vi "Main.vi"(8 "error in":errorcluster, 11 "gRPC Server Tester in":refnum<class "gRPC Server Tester.lvclass">) -> (0 "error out":errorcluster, 3 "gRPC Server Tester out":refnum<class "gRPC Server Tester.lvclass">)   [LabVIEW 2019, in "gRPC Server Tester.lvclass"]
doc: "The <b>Queued Message Handler</b> of the Worker that owns this VI."
uses:
  gRPC Server Tester.lvclass
  C:/Program Files (x86)/National Instruments/LabVIEW 2019/vi.lib/addons/_Workers/Library/Classes/Worker/Worker.lvclass
  Generated_server/RPC Messages/w4lvgrpc_Msg_ToClient_4.ctl
  Generated_server/RPC Messages/w4lvgrpc_Msg_ToClient_1.ctl
  Generated_server/RPC Messages/w4lvgrpc_Msg_ToClient_2.ctl
  Generated_server/RPC Messages/w4lvgrpc_Msg_ToClient_3.ctl
  Generated_server/RPC Messages/w4lvgrpc_Msg_ToClient_5.ctl
  Generated_server/RPC Messages/w4lvgrpc_Msg_ToServer_1.ctl
  Generated_server/RPC Messages/w4lvgrpc_Msg_ToServer_2.ctl
  Generated_server/RPC Messages/w4lvgrpc_Msg_ToServer_3.ctl
  Generated_server/RPC Messages/w4lvgrpc_Msg_ToServer_4.ctl
  Generated_server/RPC Messages/w4lvgrpc_Msg_ToServer_5.ctl
  gRPC Server Tester.lvclass/gRPC Server Tester.ctl
  gRPC Server/gRPC Server/rqp_Msg_ToClient_1.ctl
  gRPC Server/gRPC Server/rqp_Msg_ToClient_2.ctl
  gRPC Server/gRPC Server/rqp_Msg_ToClient_3.ctl
  gRPC Server/gRPC Server/rqp_Msg_ToClient_4.ctl
  gRPC Server/gRPC Server/rqp_Msg_ToClient_5.ctl
  Initialization Data.ctl
  Response Cases.ctl
  rql_Create gRPC Server.ctl
  gRPC Server/gRPC Server/rwr_Create gRPC Server.ctl
  rql_Destroy gRPC Server.ctl
  <vilib>/addons/_Workers/Library/Classes/Message Queue/Message Queue.lvclass
  gRPC Server/gRPC Server/gRPC Server.lvclass
  Generated_server/Generated_server.lvlib
panel:
  out "Msg_ToServer_5":T1
  out "Msg_ToServer_4":T2
  out "Msg_ToServer_3":T3
  out "Msg_ToServer_2":T4
  out "Msg_ToServer_1":T5
  in  "Msg_ToClient_5":T6
  in  "Msg_ToClient_3":T7
  in  "Msg_ToClient_2":T8
  in  "Msg_ToClient_1":T9
  in  "Msg_ToClient_4":T10
  out "Client ID":u64
  out "Client Connected":bool
  out "Listening Port":i32
  out "Server Listening":bool
  in  "Server Address":string="localhost:50070"
  in  "Destroy gRPC Server":bool
  in  "Create gRPC Server":bool
  # "gRPC Server Worker - Public Requests"
  # "Messages Server -> Client"
  # "gRPC Server Worker Template Example"
  # "Instructions:\n\nSee project file called Readme.md"
  # "gRPC Server Worker - Public Responses"
  # "Messages Client -> Server"
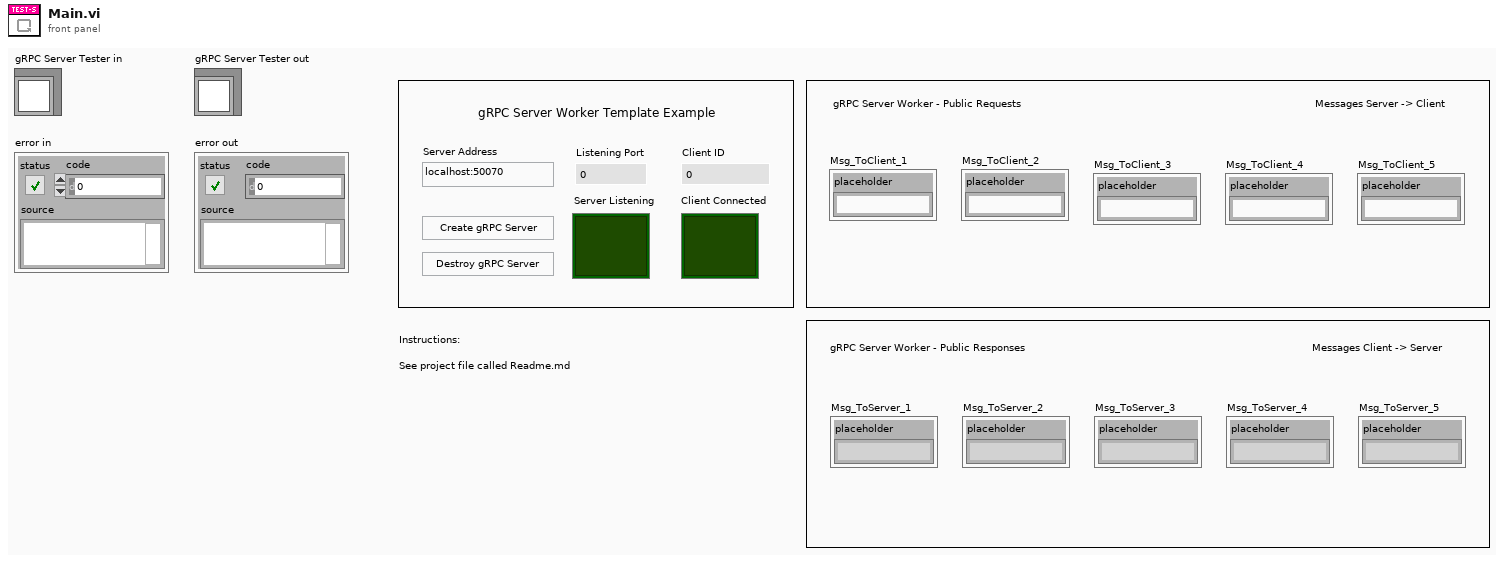
[diagram p1: front panel]
types:
  T1 = typedef "Generated_server.lvlib/w4lvgrpc_Msg_ToServer_5.ctl" = cluster{"placeholder":string}
  T2 = typedef "Generated_server.lvlib/w4lvgrpc_Msg_ToServer_4.ctl" = cluster{"placeholder":string}
  T3 = typedef "Generated_server.lvlib/w4lvgrpc_Msg_ToServer_3.ctl" = cluster{"placeholder":string}
  T4 = typedef "Generated_server.lvlib/w4lvgrpc_Msg_ToServer_2.ctl" = cluster{"placeholder":string}
  T5 = typedef "Generated_server.lvlib/w4lvgrpc_Msg_ToServer_1.ctl" = cluster{"placeholder":string}
  T6 = typedef "Generated_server.lvlib/w4lvgrpc_Msg_ToClient_5.ctl" = cluster{"placeholder":string}
  T7 = typedef "Generated_server.lvlib/w4lvgrpc_Msg_ToClient_3.ctl" = cluster{"placeholder":string}
  T8 = typedef "Generated_server.lvlib/w4lvgrpc_Msg_ToClient_2.ctl" = cluster{"placeholder":string}
  T9 = typedef "Generated_server.lvlib/w4lvgrpc_Msg_ToClient_1.ctl" = cluster{"placeholder":string}
  T10 = typedef "Generated_server.lvlib/w4lvgrpc_Msg_ToClient_4.ctl" = cluster{"placeholder":string}
  T11 = typedef "gRPC Server Tester.lvclass/Initialization Data.ctl" = cluster{"Response Cases":T12}
  T12 = typedef "gRPC Server Tester.lvclass/Response Cases.ctl" = cluster{"Placeholder - Can be deleted":string}
  T13 = typedef "gRPC Server Tester.lvclass/rql_Create gRPC Server.ctl" = cluster{"String":string}
  T14 = typedef "gRPC Server (template.proto).lvlib/gRPC Server.lvclass/rwr_Create gRPC Server.ctl" = cluster{"Server Key File (.key)":path, "Server Certificate File (.crt)":path, "Server Address":string}
  T15 = typedef "gRPC Server Tester.lvclass/rql_Destroy gRPC Server.ctl" = cluster{"String":string}
  T16 = typedef "gRPC Server (template.proto).lvlib/gRPC Server.lvclass/rqp_Msg_ToClient_1.ctl" = cluster{"w4lvgrpc_Msg_ToClient_1":T9}
  T17 = typedef "gRPC Server (template.proto).lvlib/gRPC Server.lvclass/rqp_Msg_ToClient_2.ctl" = cluster{"w4lvgrpc_Msg_ToClient_2":T8}
  T18 = typedef "gRPC Server (template.proto).lvlib/gRPC Server.lvclass/rqp_Msg_ToClient_3.ctl" = cluster{"w4lvgrpc_Msg_ToClient_3":T7}
  T19 = typedef "gRPC Server (template.proto).lvlib/gRPC Server.lvclass/rqp_Msg_ToClient_4.ctl" = cluster{"w4lvgrpc_Msg_ToClient_4":T10}
  T20 = typedef "gRPC Server (template.proto).lvlib/gRPC Server.lvclass/rqp_Msg_ToClient_5.ctl" = cluster{"w4lvgrpc_Msg_ToClient_5":T6}
  T21 = typedef "gRPC Server (template.proto).lvlib/gRPC Server.lvclass/rwr_Create gRPC Server Reply.ctl" = cluster{"Listening Port":i32}
  T22 = typedef "gRPC Server (template.proto).lvlib/gRPC Server.lvclass/rsp_Connection Notify.ctl" = cluster{"gRPC ID":T23, "Connected?":bool}
  T23 = typedef "grpc-lvsupport-release.lvlib/grpcId.ctl" = u64
  T24 = typedef "gRPC Server (template.proto).lvlib/gRPC Server.lvclass/rsp_Server Error.ctl" = errorcluster
  T25 = typedef "gRPC Server (template.proto).lvlib/gRPC Server.lvclass/rsp_Msg_ToServer_1.ctl" = cluster{"w4lvgrpc_Msg_ToServer_1":T5}
  T26 = typedef "gRPC Server (template.proto).lvlib/gRPC Server.lvclass/rsp_Msg_ToServer_2.ctl" = cluster{"w4lvgrpc_Msg_ToServer_2":T4}
  T27 = typedef "gRPC Server (template.proto).lvlib/gRPC Server.lvclass/rsp_Msg_ToServer_3.ctl" = cluster{"w4lvgrpc_Msg_ToServer_3":T3}
  T28 = typedef "gRPC Server (template.proto).lvlib/gRPC Server.lvclass/rsp_Msg_ToServer_4.ctl" = cluster{"w4lvgrpc_Msg_ToServer_4":T2}
  T29 = typedef "gRPC Server (template.proto).lvlib/gRPC Server.lvclass/rsp_Msg_ToServer_5.ctl" = cluster{"w4lvgrpc_Msg_ToServer_5":T1}
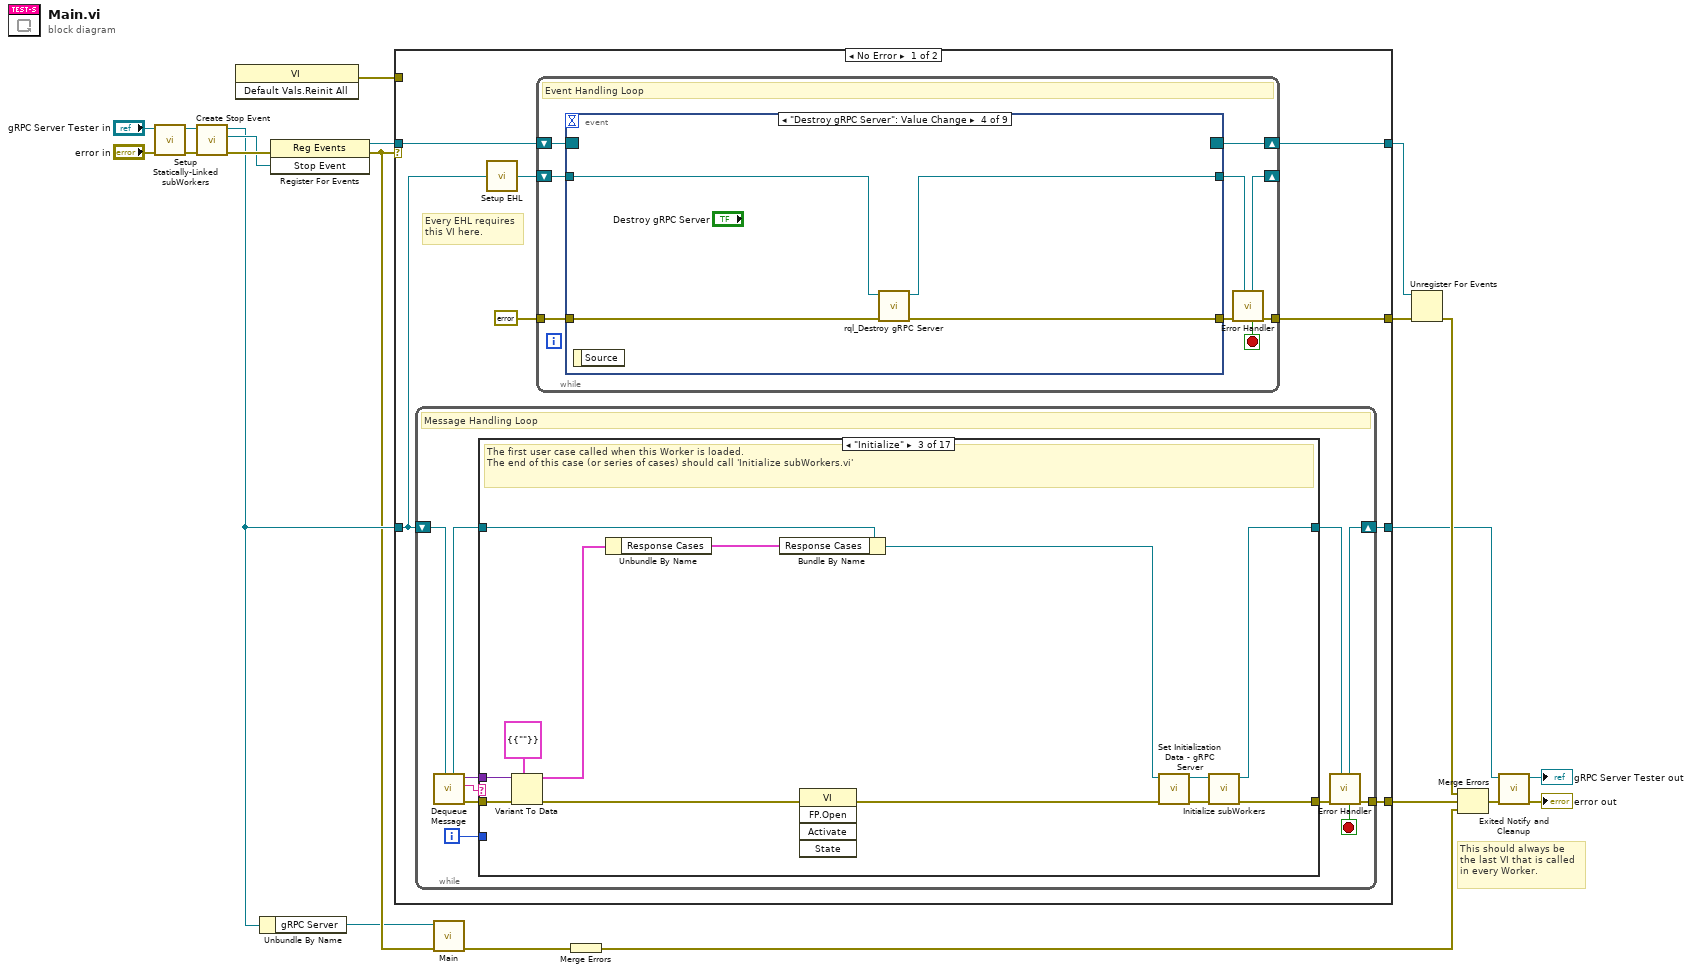
[diagram p0: block diagram]
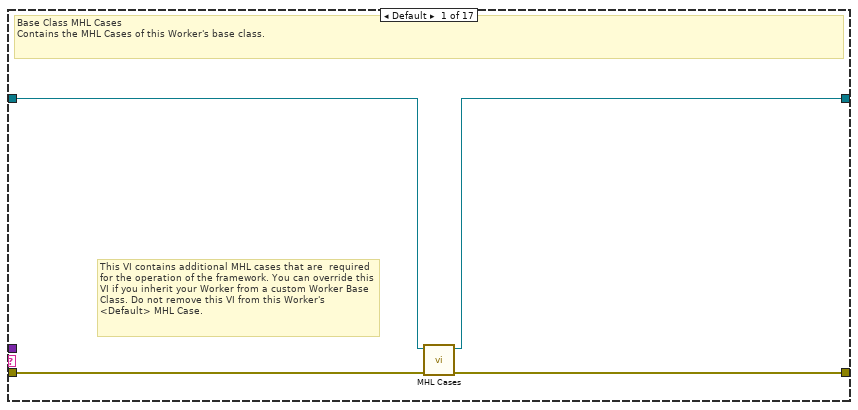
[diagram p2: hidden frame]
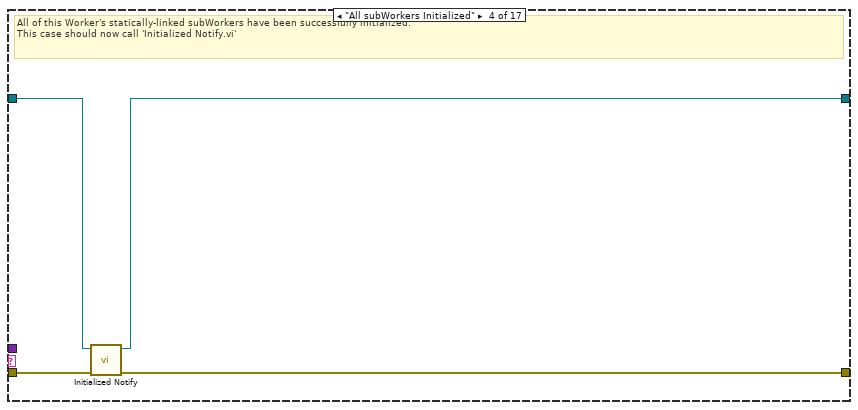
[diagram p4: hidden frame]
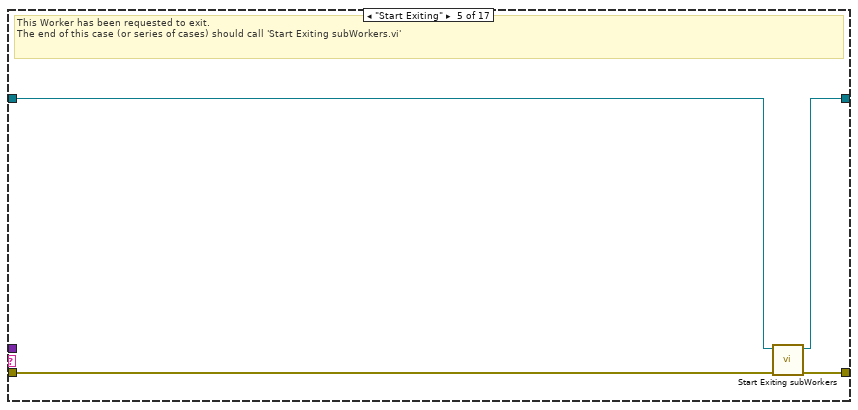
[diagram p5: hidden frame]
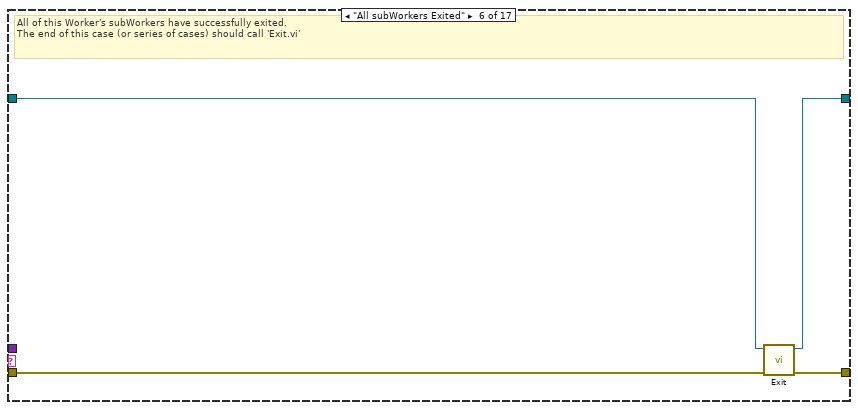
[diagram p6: hidden frame]
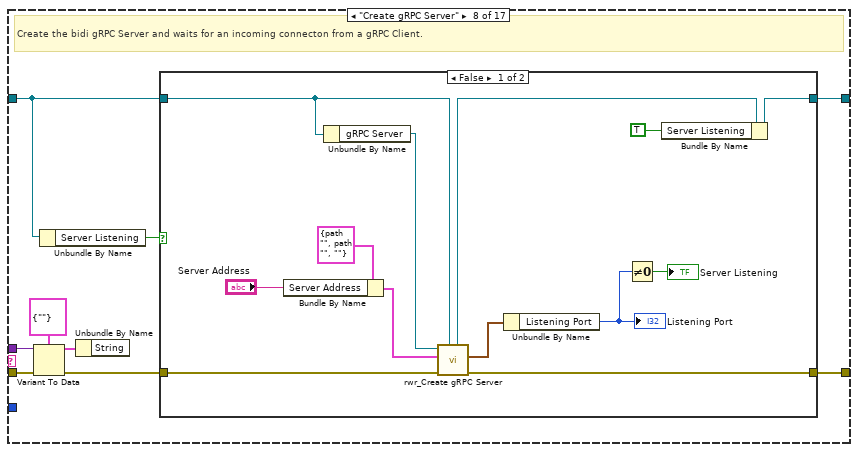
[diagram p8: hidden frame]
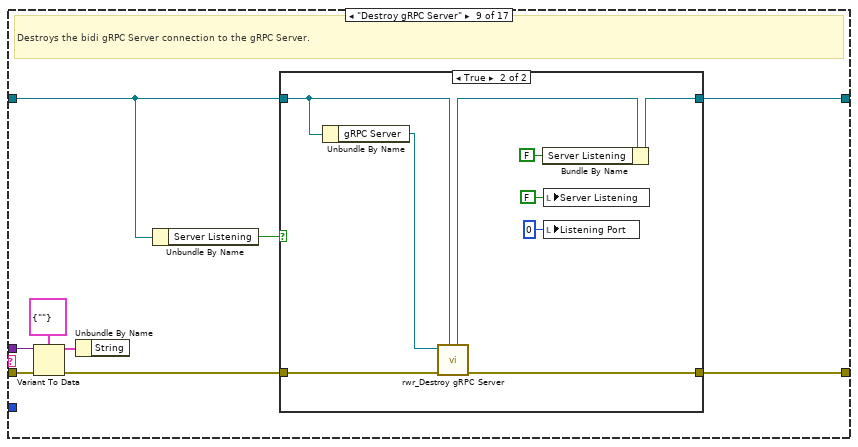
[diagram p10: hidden frame]
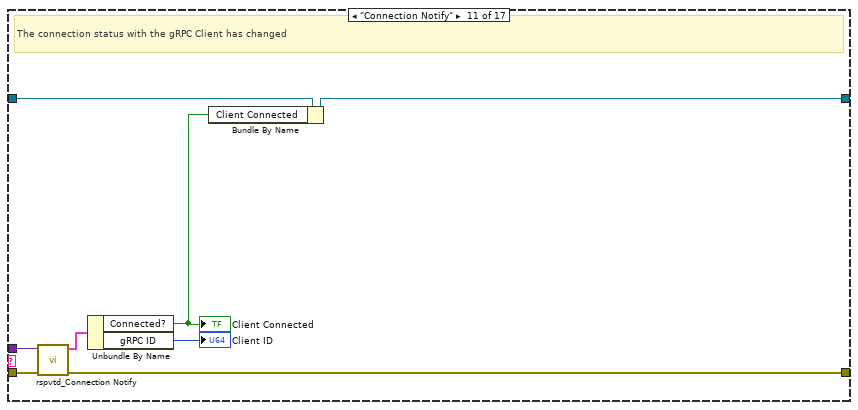
[diagram p13: hidden frame]
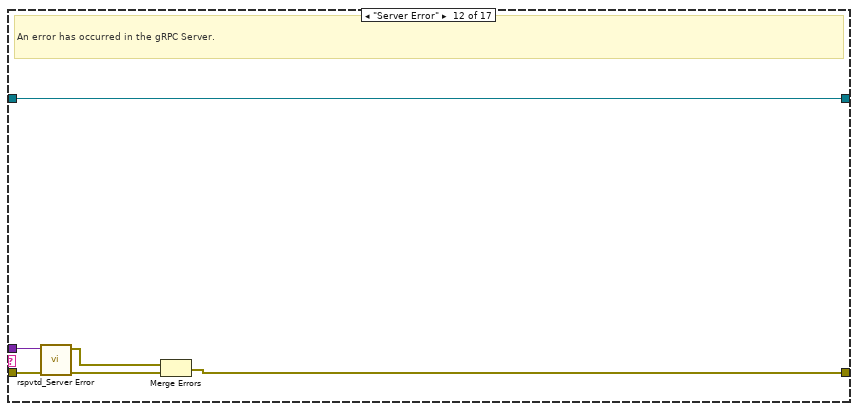
[diagram p14: hidden frame]
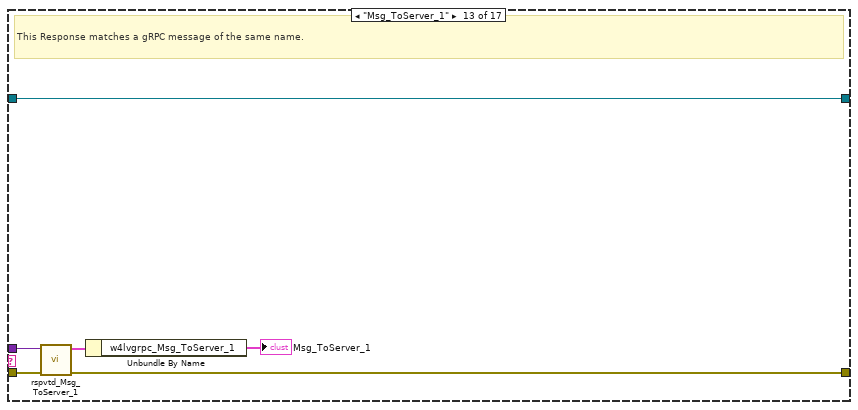
[diagram p15: hidden frame]
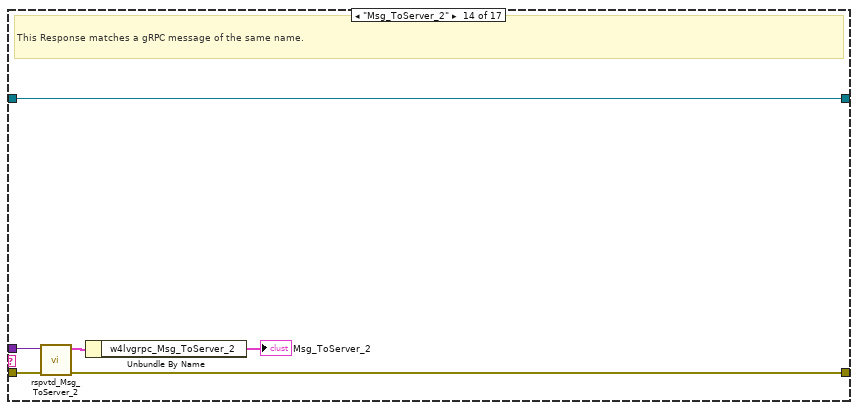
[diagram p16: hidden frame]
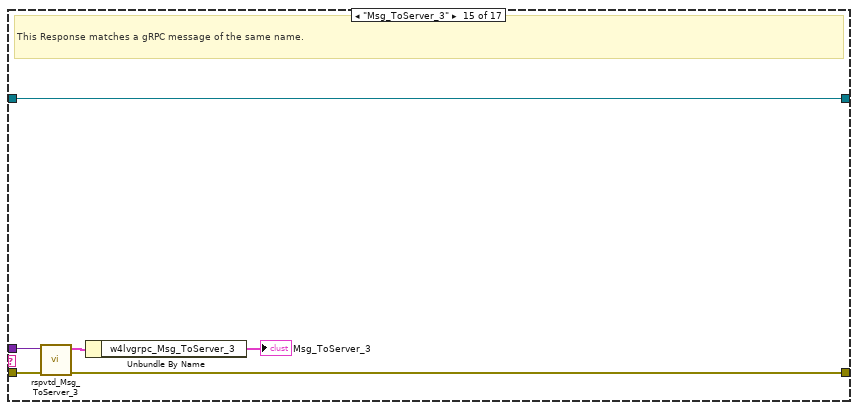
[diagram p17: hidden frame]
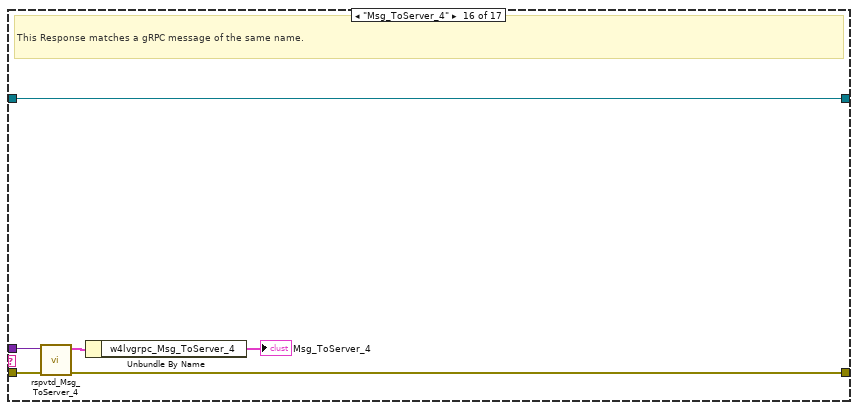
[diagram p18: hidden frame]
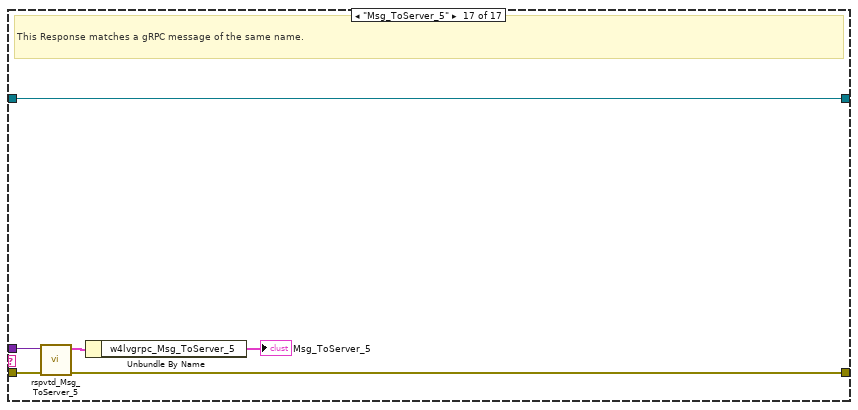
[diagram p19: hidden frame]
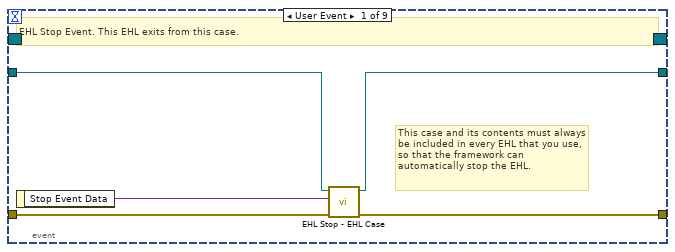
[diagram p20: hidden frame]
diagram:
  # "This should always be the last VI that is called in every Worker."
  n1 = call "Setup Statically-Linked subWorkers.vi"("error in"="error in", "gRPC Server Tester in"="gRPC Server Tester in") -> ("error out"=w7:errorcluster, "gRPC Server Tester out"=w5:refnum<class "gRPC Server Tester.lvclass">)  [unwired: 8 in]
  n2 = call-dynamic "Create Stop Event.vi"("error in"=w7, "Worker"=w5) -> ("error out"=w16:errorcluster, "Stop Event"=w13:refnum<user-event>, "Worker out"=w10:refnum<class "gRPC Server Tester.lvclass">)  [unwired: 7 in]
  n3 = invoke class="VI" method="Default Vals.Reinit All"() -> (error out=w1:errorcluster)  [unwired: 3 in, 2 out]
  n4 = Unbundle By Name(w10) -> ("gRPC Server"=w2:refnum<class "gRPC Server.lvclass">)
  n5 = register-events(error in=w16, w13) -> (reference out=w15:refnum<event-registration>, error out=w8:errorcluster)  [unwired: 1 in]
  n6 = case shown="No Error" w8 {
    tunnel: w10 -> [w24 w234]
    tunnel: [w22 w235] -> w14
    tunnel: w15 -> [w29 w236]
    tunnel: [w26 w237] -> w20
    tunnel: [w28 w236] -> w19
    tunnel: [w23 w233] -> w17
    selector: w8 -> [_ w237]
    tunnel: w1 -> [_ _]
    frame No Error {
      # "Every EHL requires\nthis VI here."
      n7 = while {
        shift-right: [w38] -> w23
        shift-left: w24 -> [w40]
        tunnel: [w39] -> w22
        i -> [w31]
        stop <- w32 stop-if-true
        # "Message Handling Loop"
        n8 = call-dynamic "Dequeue Message.vi"("Worker"=w40) -> ("error out"=w37:errorcluster, "Case out"=w33:string, "Data out"=w30:variant, "Worker out"=w35:refnum<class "gRPC Server Tester.lvclass">)  [unwired: 6 in, 1 out]
        n9 = case "Worker MHL Case Structure (DO NOT CHANGE LABEL NAME)" shown="\"Initialize\"" w33 {
          tunnel: w37 -> [w44 w45 w57 w62 w64 w71 w73 w82 w106 w119 w127 w133 w139 w145 w151 w157 w163]
          tunnel: [w43 w45 w59 w60 w67 w70 w73 w77 w101 w119 w120 w129 w137 w143 w149 w155 w161] -> w36
          tunnel: w35 -> [w42 w46 w56 w63 w65 w69 w72 w75 w99 w118 w126 w132 w138 w144 w150 w156 w162]
          tunnel: [w41 w46 w58 w61 w66 w68 w72 w76 w100 w118 w121 w132 w138 w144 w150 w156 w162] -> w34
          tunnel: w31 -> [_ _ _ _ _ _ _ _ _ _ _ _ _ _ _ _ _]
          tunnel: w30 -> [_ _ w55 _ _ _ _ w79 w103 _ w125 w130 w136 w142 w148 w154 w160]
          frame Default {
            # "This VI contains additional MHL cases that are  required for the operation of the framework. You can override this VI if you inherit your Worker from a custom Worker Base Class. Do not remove this VI from this Worker's <Default> MHL Case."
            # "Base Class MHL Cases\nContains the MHL Cases of this Worker's base class."
            n10 = call-dynamic "MHL Cases.vi"("error in"=w44, "Worker in"=w42) -> ("error out"=w43:errorcluster, "Worker out"=w41:refnum<class "gRPC Server Tester.lvclass">)  [unwired: 8 in]
          }
          frame "------------ FRAMEWORK CASES -----------" {
            # "Start of Workers Framework Cases"
          }
          frame "Initialize" {
            # "The first user case called when this Worker is loaded.\nThe end of this case (or series of cases) should call 'Initialize subWorkers.vi'"
            n11 = Variant To Data(error in=w57, type=T11 {"Response Cases"={"Placeholder - Can be deleted"=""}} ("Initialization Data"), Variant=w55) -> (data=w54:T11, error out=w48:errorcluster)
            n12 = Unbundle By Name(w54) -> ("Response Cases"=w53:T12)
            n13 = Bundle By Name(cluster=w56, "Response Cases"=w53) -> (w49:refnum<class "gRPC Server Tester.lvclass">)
            n14 = invoke class="VI" method="FP.Open"(error in=w48) -> (error out=w47:errorcluster)  [unwired: 4 in, 4 out]
            n15 = call "Set Initialization Data - gRPC Server.vi"("error in"=w47, "gRPC Server Tester in"=w49) -> ("error out"=w51:errorcluster, "gRPC Server Tester out"=w50:refnum<class "gRPC Server Tester.lvclass">)  [unwired: 8 in]
            n16 = call-dynamic "Initialize subWorkers.vi"("error in"=w51, "Worker"=w50) -> ("error out"=w59:errorcluster, "dup Worker out"=w58:refnum<class "gRPC Server Tester.lvclass">)  [unwired: 8 in]
          }
          frame "All subWorkers Initialized" {
            # "All of this Worker's statically-linked subWorkers have been successfully initialized.\nThis case should now call 'Initialized Notify.vi'"
            n17 = call-dynamic "Initialized Notify.vi"("error in"=w62, "Worker"=w63) -> ("error out"=w60:errorcluster, "dup Worker out"=w61:refnum<class "gRPC Server Tester.lvclass">)  [unwired: 8 in]
          }
          frame "Start Exiting" {
            # "This Worker has been requested to exit. \nThe end of this case (or series of cases) should call 'Start Exiting subWorkers.vi'"
            n18 = call-dynamic "Start Exiting subWorkers.vi"("error_in"=w64, "Worker"=w65) -> ("error out"=w67:errorcluster, "dup Worker out"=w66:refnum<class "gRPC Server Tester.lvclass">)  [unwired: 8 in]
          }
          frame "All subWorkers Exited" {
            # "All of this Worker's subWorkers have successfully exited. \nThe end of this case (or series of cases) should call 'Exit.vi'"
            n19 = call-dynamic "Exit.vi"("error_in"=w71, "Worker"=w69) -> ("error out"=w70:errorcluster, "dup Worker out"=w68:refnum<class "gRPC Server Tester.lvclass">)  [unwired: 8 in]
          }
          frame "------------- LOCAL API CASES -------------" {
            # "Start of Workers Local API Cases"
          }
          frame "Create gRPC Server" {
            # "Create the bidi gRPC Server and waits for an incoming connecton from a gRPC Client."
            n20 = Variant To Data(error in=w82, type=T13 {"String"=""} ("Data"), Variant=w79) -> (data=w78:T13, error out=w81:errorcluster)
            n21 = Unbundle By Name(w75) -> ("Server Listening"=w74:bool)
            n22 = Unbundle By Name(w78) -> ()  [unwired: 1 out]
            n23 = case shown="False" w74 {
              tunnel: w81 -> [w95 w96]
              tunnel: [w94 w96] -> w77
              tunnel: [w84 w97] -> w76
              tunnel: w75 -> [w92 w97]
              frame False {
                n24 = Bundle By Name(cluster=T14 {"Server Key File (.key)"=path "", "Server Certificate File (.crt)"=path "", "Server Address"=""} ("Data in"), "Server Address"="Server Address") -> (w89:T14)
                n25 = Unbundle By Name(w92) -> ("gRPC Server"=w91:refnum<class "gRPC Server.lvclass">)
                n26 = call "rwr_Create gRPC Server.vi"("Caller in"=w92, "error in"=w95, "Data in"=w89, "gRPC Server in"=w91) -> ("error out"=w94:errorcluster, "Reply Data out"=w87:T21, "dup Caller out"=w93:refnum<class "gRPC Server Tester.lvclass">)  [unwired: 4 in, 1 out]
                n27 = Unbundle By Name(w87) -> ("Listening Port"=w86:i32)
                "Listening Port" <- w86
                n28 = Not Equal To 0?(x=w86) -> (x != 0?=→"Server Listening":bool)
                n29 = Bundle By Name(cluster=w93, "Server Listening"=TRUE) -> (w84:refnum<class "gRPC Server Tester.lvclass">)
              }
              frame True {
                # "Already listening. Nothing to do."
              }
            }
          }
          frame "Destroy gRPC Server" {
            # "Destroys the bidi gRPC Server connection to the gRPC Server."
            n30 = Variant To Data(error in=w106, type=T15 {"String"=""} ("Data"), Variant=w103) -> (data=w102:T15, error out=w105:errorcluster)
            n31 = Unbundle By Name(w102) -> ()  [unwired: 1 out]
            n32 = Unbundle By Name(w99) -> ("Server Listening"=w98:bool)
            n33 = case shown="True" w98 {
              tunnel: w105 -> [w107 w117]
              tunnel: [w107 w112] -> w101
              tunnel: [w108 w113] -> w100
              tunnel: w99 -> [w108 w115]
              frame False {
                # "Server not listening. Nothing to do"
              }
              frame True {
                n34 = Unbundle By Name(w115) -> ("gRPC Server"=w114:refnum<class "gRPC Server.lvclass">)
                n35 = call "rwr_Destroy gRPC Server.vi"("Caller in"=w115, "error in"=w117, "gRPC Server in"=w114) -> ("error out"=w112:errorcluster, "dup Caller out"=w116:refnum<class "gRPC Server Tester.lvclass">)  [unwired: 5 in, 2 out]
                n36 = Bundle By Name(cluster=w116, "Server Listening"=FALSE) -> (w113:refnum<class "gRPC Server Tester.lvclass">)
                n37 = local write "Server Listening"(FALSE ("Server Listening")) -> ()
                n38 = local write "Listening Port"(0 ("Listening Port")) -> ()
              }
            }
          }
          frame "------------- RESPONSE CASES --------------" {
            # "Start of Workers Response Cases"
          }
          frame "Connection Notify" {
            # "The connection status with the gRPC Client has changed"
            n39 = call "rspvtd_Connection Notify.vi"("error in"=w127, "Data in"=w125) -> ("error out"=w120:errorcluster, "Data out"=w124:T22)  [unwired: 8 in]
            n40 = Unbundle By Name(w124) -> ("Connected?"=w123:bool, "gRPC ID"=→"Client ID":T23)
            "Client Connected" <- w123
            n41 = Bundle By Name(cluster=w126, "Client Connected"=w123) -> (w121:refnum<class "gRPC Server Tester.lvclass">)
          }
          frame "Server Error" {
            # "An error has occurred in the gRPC Server."
            n42 = call "rspvtd_Server Error.vi"("error in"=w133, "Data in"=w130) -> ("error out"=w131:errorcluster, "Data out"=w128:T24)  [unwired: 8 in]
            n43 = Merge Errors(w128, w131) -> (w129:errorcluster)
          }
          frame "Msg_ToServer_1" {
            # "This Response matches a gRPC message of the same name."
            n44 = call "rspvtd_Msg_ToServer_1.vi"("error in"=w139, "Data in"=w136) -> ("error out"=w137:errorcluster, "Data out"=w135:T25)  [unwired: 8 in]
            n45 = Unbundle By Name(w135) -> ("w4lvgrpc_Msg_ToServer_1"=→"Msg_ToServer_1":T5)
          }
          frame "Msg_ToServer_2" {
            # "This Response matches a gRPC message of the same name."
            n46 = call "rspvtd_Msg_ToServer_2.vi"("error in"=w145, "Data in"=w142) -> ("error out"=w143:errorcluster, "Data out"=w141:T26)  [unwired: 8 in]
            n47 = Unbundle By Name(w141) -> ("w4lvgrpc_Msg_ToServer_2"=→"Msg_ToServer_2":T4)
          }
          frame "Msg_ToServer_3" {
            # "This Response matches a gRPC message of the same name."
            n48 = call "rspvtd_Msg_ToServer_3.vi"("error in"=w151, "Data in"=w148) -> ("error out"=w149:errorcluster, "Data out"=w147:T27)  [unwired: 8 in]
            n49 = Unbundle By Name(w147) -> ("w4lvgrpc_Msg_ToServer_3"=→"Msg_ToServer_3":T3)
          }
          frame "Msg_ToServer_4" {
            # "This Response matches a gRPC message of the same name."
            n50 = call "rspvtd_Msg_ToServer_4.vi"("error in"=w157, "Data in"=w154) -> ("error out"=w155:errorcluster, "Data out"=w153:T28)  [unwired: 8 in]
            n51 = Unbundle By Name(w153) -> ("w4lvgrpc_Msg_ToServer_4"=→"Msg_ToServer_4":T2)
          }
          frame "Msg_ToServer_5" {
            # "This Response matches a gRPC message of the same name."
            n52 = call "rspvtd_Msg_ToServer_5.vi"("error in"=w163, "Data in"=w160) -> ("error out"=w161:errorcluster, "Data out"=w159:T29)  [unwired: 8 in]
            n53 = Unbundle By Name(w159) -> ("w4lvgrpc_Msg_ToServer_5"=→"Msg_ToServer_5":T1)
          }
        }
        n54 = call-dynamic "Error Handler.vi"("Worker"=w34, "error_in"=w36) -> ("error out"=w39:errorcluster, "Stop Loop"=w32:bool, "Worker out"=w38:refnum<class "gRPC Server Tester.lvclass">)  [unwired: 7 in]
      }
      n55 = call-dynamic "Setup EHL.vi"("Worker"=w24) -> ("Worker out"=w25:refnum<class "gRPC Server Tester.lvclass">)  [unwired: 14 in]
      n56 = while "Event Handling Loop" {
        shift-right: [w172] -> w28
        shift-left: w29 -> [w171]
        tunnel: [w167] -> w26
        tunnel: errorcluster {"status"=FALSE, "code"=0, "source"=""} ("error constant") -> [w169]
        shift-right: [w165] -> _
        shift-left: w25 -> [w170]
        stop <- w164 stop-if-true
        # "Event Handling Loop"
        n57 = event shown="[3] \"Destroy gRPC Server\": Value Change" {
          selector: w171 -> [_ _ _ _ _ _ _ _ _]
          dyn-events: [_ _ _ _ _ _ _ _ _] -> w172
          timeout: _ -> [_ _ _ _ _ _ _ _ _]
          tunnel: [w176 w183 w187 w191 w199 w207 w215 w223 w231] -> w168
          tunnel: w169 -> [w177 w182 w188 w192 w200 w208 w216 w224 w232]
          tunnel: w170 -> [w175 w181 w186 w190 w195 w203 w211 w219 w227]
          tunnel: [w174 w180 w185 w189 w198 w206 w214 w222 w230] -> w166
          event User Event {
            # "This case and its contents must always be included in every EHL that you use, so that the framework can automatically stop the EHL."
            # "EHL Stop Event. This EHL exits from this case."
            n58 = event-data() -> ("Stop Event Data"=w173:variant)  [unwired: 1 in]
            n59 = call-dynamic "EHL Stop - EHL Case.vi"("error in"=w177, "Stop Event Data"=w173, "Worker"=w175) -> ("error out"=w176:errorcluster, "Worker out"=w174:refnum<class "gRPC Server Tester.lvclass">)  [unwired: 7 in]
          }
          event Panel Close? {
            # "Use this VI when you want to exit this Worker. This VI will call the Start Exiting case of this Worker. This is the correct way to exit your Worker."
            # "Calls the Start Exiting case of this Worker. This will start the exiting sequence of this Worker."
            n60 = event-data() -> ()  [unwired: 1 in, 1 out]
            n61 = property class="gRPC Server Tester"(reference=w181) -> (reference out=w179:refnum<class "gRPC Server Tester.lvclass">, "Accessors:Read:Public API:Queue"=w178:refnum<class "Message Queue.lvclass">)  [unwired: 1 in, 1 out]
            n62 = call-dynamic "Worker Start Exiting.vi"("error_in"=w182, "Message Queue"=w178, "Worker"=w179) -> ("error out"=w183:errorcluster, "dup Worker out"=w180:refnum<class "gRPC Server Tester.lvclass">)  [unwired: 7 in]
            n63 = event-data ("Event Filter Node")("Discard?"=TRUE) -> ()  [unwired: 1 in, 1 out]
          }
          event "Create gRPC Server": Value Change {
            n64 = event-data() -> ()  [unwired: 1 in, 1 out]
            n65 = call "rql_Create gRPC Server.vi"("error in"=w188, "gRPC Server Tester in"=w186) -> ("error out"=w187:errorcluster, "dup gRPC Server Tester out"=w185:refnum<class "gRPC Server Tester.lvclass">)  [unwired: 8 in]
          }
          event "Destroy gRPC Server": Value Change {
            n66 = event-data() -> ()  [unwired: 1 in, 1 out]
            n67 = call "rql_Destroy gRPC Server.vi"("error in"=w192, "gRPC Server Tester in"=w190) -> ("error out"=w191:errorcluster, "dup gRPC Server Tester out"=w189:refnum<class "gRPC Server Tester.lvclass">)  [unwired: 8 in]
          }
          event Value Change {
            n68 = event-data() -> ()  [unwired: 1 in, 1 out]
            n69 = Bundle By Name(cluster=T16 {"w4lvgrpc_Msg_ToClient_1"={"placeholder"=""}} ("Data in"), "w4lvgrpc_Msg_ToClient_1"="Msg_ToClient_1") -> (w196:T16)
            n70 = Unbundle By Name(w195) -> ("gRPC Server"=w194:refnum<class "gRPC Server.lvclass">)
            n71 = call "rqp_Msg_ToClient_1.vi"("Caller in"=w195, "error in"=w200, "Data in"=w196, "gRPC Server in"=w194) -> ("error out"=w199:errorcluster, "dup Caller out"=w198:refnum<class "gRPC Server Tester.lvclass">)  [unwired: 5 in, 1 out]
          }
          event Value Change {
            n72 = event-data() -> ()  [unwired: 1 in, 1 out]
            n73 = Bundle By Name(cluster=T17 {"w4lvgrpc_Msg_ToClient_2"={"placeholder"=""}} ("Data in"), "w4lvgrpc_Msg_ToClient_2"="Msg_ToClient_2") -> (w204:T17)
            n74 = Unbundle By Name(w203) -> ("gRPC Server"=w202:refnum<class "gRPC Server.lvclass">)
            n75 = call "rqp_Msg_ToClient_2.vi"("Caller in"=w203, "error in"=w208, "Data in"=w204, "gRPC Server in"=w202) -> ("error out"=w207:errorcluster, "dup Caller out"=w206:refnum<class "gRPC Server Tester.lvclass">)  [unwired: 5 in, 1 out]
          }
          event Value Change {
            n76 = event-data() -> ()  [unwired: 1 in, 1 out]
            n77 = Bundle By Name(cluster=T18 {"w4lvgrpc_Msg_ToClient_3"={"placeholder"=""}} ("Data in"), "w4lvgrpc_Msg_ToClient_3"="Msg_ToClient_3") -> (w212:T18)
            n78 = Unbundle By Name(w211) -> ("gRPC Server"=w210:refnum<class "gRPC Server.lvclass">)
            n79 = call "rqp_Msg_ToClient_3.vi"("Caller in"=w211, "error in"=w216, "Data in"=w212, "gRPC Server in"=w210) -> ("error out"=w215:errorcluster, "dup Caller out"=w214:refnum<class "gRPC Server Tester.lvclass">)  [unwired: 5 in, 1 out]
          }
          event Value Change {
            n80 = event-data() -> ()  [unwired: 1 in, 1 out]
            n81 = Bundle By Name(cluster=T19 {"w4lvgrpc_Msg_ToClient_4"={"placeholder"=""}} ("Data in"), "w4lvgrpc_Msg_ToClient_4"="Msg_ToClient_4") -> (w220:T19)
            n82 = Unbundle By Name(w219) -> ("gRPC Server"=w218:refnum<class "gRPC Server.lvclass">)
            n83 = call "rqp_Msg_ToClient_4.vi"("Caller in"=w219, "error in"=w224, "Data in"=w220, "gRPC Server in"=w218) -> ("error out"=w223:errorcluster, "dup Caller out"=w222:refnum<class "gRPC Server Tester.lvclass">)  [unwired: 5 in, 1 out]
          }
          event Value Change {
            n84 = event-data() -> ()  [unwired: 1 in, 1 out]
            n85 = Bundle By Name(cluster=T20 {"w4lvgrpc_Msg_ToClient_5"={"placeholder"=""}} ("Data in"), "w4lvgrpc_Msg_ToClient_5"="Msg_ToClient_5") -> (w228:T20)
            n86 = Unbundle By Name(w227) -> ("gRPC Server"=w226:refnum<class "gRPC Server.lvclass">)
            n87 = call "rqp_Msg_ToClient_5.vi"("Caller in"=w227, "error in"=w232, "Data in"=w228, "gRPC Server in"=w226) -> ("error out"=w231:errorcluster, "dup Caller out"=w230:refnum<class "gRPC Server Tester.lvclass">)  [unwired: 5 in, 1 out]
          }
        }
        n88 = call-dynamic "Error Handler.vi"("Worker"=w166, "error_in"=w168) -> ("error out"=w167:errorcluster, "Stop Loop"=w164:bool, "Worker out"=w165:refnum<class "gRPC Server Tester.lvclass">)  [unwired: 7 in]
      }
    }
    frame Error {
      n89 = call-dynamic "Error Handler.vi"("Worker"=w234, "error_in"=w237) -> ("error out"=w235:errorcluster, "Worker out"=w233:refnum<class "gRPC Server Tester.lvclass">)  [unwired: 7 in, 1 out]
    }
  }
  n90 = call-dynamic "Main.vi"("error in"=w8, "gRPC Server in"=w2) -> ("error out"=w4:errorcluster)  [unwired: 8 in, 1 out]
  n91 = Merge Errors(w4) -> (w3:errorcluster)
  n92 = Unregister For Events(event registration refnum=w19, error in=w20) -> (error out=w21:errorcluster)
  n93 = Merge Errors(w21, w14, w3) -> (w18:errorcluster)
  n94 = call-dynamic "Exited Notify and Cleanup.vi"("error_in"=w18, "Worker"=w17) -> ("error out"=→"error out":errorcluster, "dup Worker out"=→"gRPC Server Tester out":refnum<class "gRPC Server Tester.lvclass">)  [unwired: 8 in]
